vi "执行校准.vi"(3 "校准点位":u16(ring) caption="校准方式：" items=["第一点校准", "第二点校准", "第三点校准"], 5 "校准方式":u16(ring) caption="校准方式：" items=["单点校准", "两点校准", "三点校准"], 6 "校准量程":u16, 7 "校准参数":u16(ring) caption="校准参数：" items=["pH", "DO", "浊度", "电导率", "叶绿素a", "藻密度", "ORP", "COD", "DO2", "氯化物", "氨氮", "水火油"], 8 "error in (no error)":errorcluster caption="错误输入（无错误）", 9 "标液三":cluster{"标准值":dbl, "检测值":dbl, "原始值":dbl} caption="标液三：" {"原始值" format="%#.6f"; "检测值" format="%#.6f"; "标准值" format="%#.6f"}, 10 "标液二":cluster{"标准值":dbl, "检测值":dbl, "原始值":dbl} caption="标液二：" {"原始值" format="%#.6f"; "检测值" format="%#.6f"; "标准值" format="%#.6f"}, 11 "标液一":cluster{"标准值":dbl, "检测值":dbl, "原始值":dbl} caption="标液一：" {"原始值" format="%#.6f"; "检测值" format="%#.6f"; "标准值" format="%#.6f"}) -> (0 "error out":errorcluster)   [LabVIEW 2016, in "斯坦道多参数.lvlib"]
panel:
  in  "选项卡控件":enum32{"选项卡 1"}(tab)
  # "检测值"
  # "原始值"
  # "标准值"
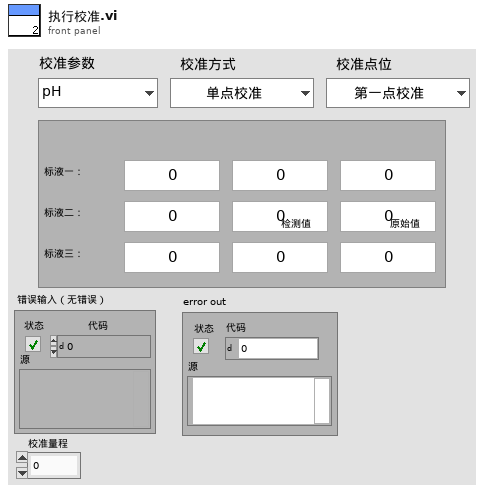
[diagram p1: front panel]
types:
  T1 = typedef "斯坦道多参数.lvlib/探头类型.ctl" = enum16{"禹山", "国弘", "纳清", "STD"}
  T2 = cluster{"pH探头选择":T1, "DO探头选择":T1, "电导率探头选择":T1, "浊度探头选择":T1, "悬浮物探头选择":T1, "叶绿素a探头选择":T1, "蓝绿藻探头选择":T1, "orp探头选择":T1, "COD探头选择":T1, "DO2探头选择":T1, "氨氮探头选择":T1, "水中油探头选择":T1, "余氯探头选择":T1}
  T3 = enum16{"NULL", "pH", "Cond", "DO", "Turb", "ORP", "6", "7", "COD", "9", "氯化物", "11", "12", "13", "14", "15", "16", "水中油"}
  T4 = enum16{"null", "pH", "DO", "浊度", "电导率", "叶绿素a", "藻密度", "氨氮"}
  T5 = enum16{"null", "pH", "DO", "浊度", "电导率", "叶绿素a", "DO2"}
  T6 = enum16{"null", "pH", "DO", "浊度", "电导率", "叶绿素a", "DO2", "藻密度"}
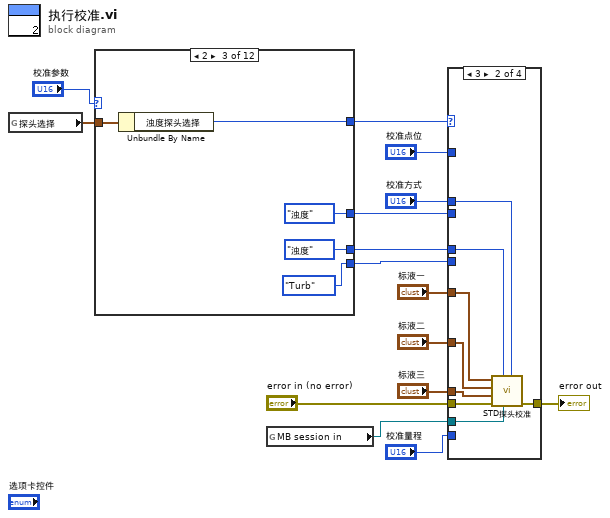
[diagram p0: block diagram]
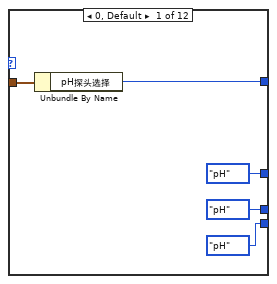
[diagram p2: hidden frame]
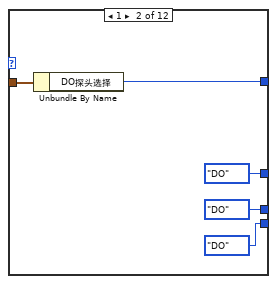
[diagram p3: hidden frame]
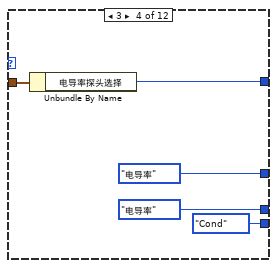
[diagram p4: hidden frame]
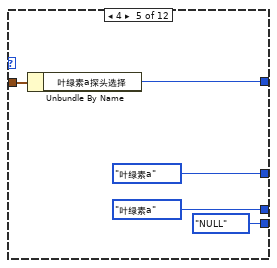
[diagram p5: hidden frame]
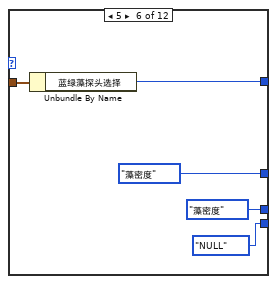
[diagram p6: hidden frame]
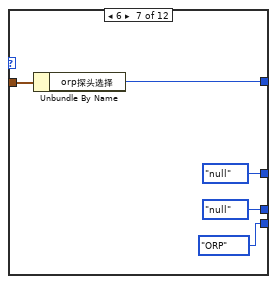
[diagram p7: hidden frame]
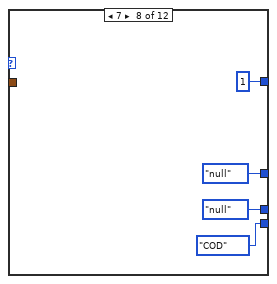
[diagram p8: hidden frame]
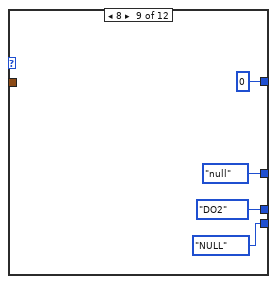
[diagram p9: hidden frame]
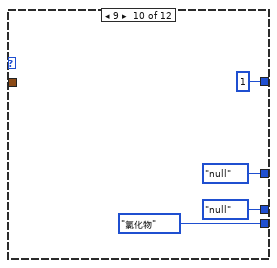
[diagram p10: hidden frame]
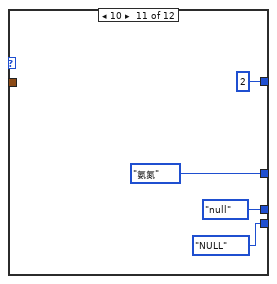
[diagram p11: hidden frame]
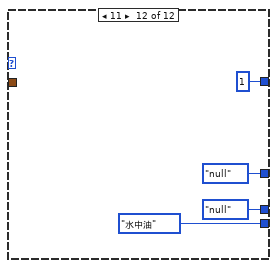
[diagram p12: hidden frame]
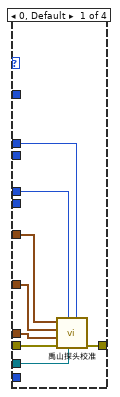
[diagram p13: hidden frame]
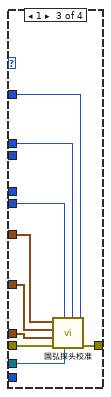
[diagram p14: hidden frame]
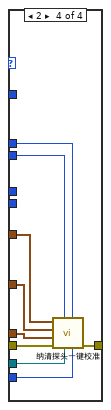
[diagram p15: hidden frame]
diagram:
  n1 = global read "断电保存变量.vi" "探头选择"() -> (w6:T2)
  n2 = case shown="2" "校准参数" {
    tunnel: [T5."pH" ("探头") T5."DO" ("探头") T5."浊度" ("探头") T5."电导率" ("探头") T5."叶绿素a" ("探头") T6."藻密度" ("探头") T5."null" ("探头") T5."null" ("探头") T5."DO2" ("探头") T5."null" ("探头") T5."null" ("探头") T5."null" ("探头")] -> w7
    tunnel: w6 -> [w19 w24 w29 w34 w40 w44 w49 _ _ _ _ _]
    tunnel: [w18 w23 w28 w33 w39 w43 w48 u16 1 ("orp探头选择") u16 0 ("orp探头选择") u16 1 ("orp探头选择") u16 2 ("orp探头选择") u16 1 ("orp探头选择")] -> w5
    tunnel: [T4."pH" ("探头") T4."DO" ("探头") T4."浊度" ("探头") T4."电导率" ("探头") T4."叶绿素a" ("探头") T4."藻密度" ("探头") T4."null" ("探头") T4."null" ("探头") T4."null" ("探头") T4."null" ("探头") T4."氨氮" ("探头") T4."null" ("探头")] -> w4
    tunnel: [T3."pH" ("探头") T3."DO" ("探头") T3."Turb" ("探头") T3."Cond" ("探头") T3."NULL" ("探头") T3."NULL" ("探头") T3."ORP" ("探头") T3."COD" ("探头") T3."NULL" ("探头") T3."氯化物" ("探头") T3."NULL" ("探头") T3."水中油" ("探头")] -> w3
    frame 0, Default {
      n3 = Unbundle By Name(w19) -> ("pH探头选择"=w18:T1)
    }
    frame 1 {
      n4 = Unbundle By Name(w24) -> ("DO探头选择"=w23:T1)
    }
    frame 2 {
      n5 = Unbundle By Name(w29) -> ("浊度探头选择"=w28:T1)
    }
    frame 3 {
      n6 = Unbundle By Name(w34) -> ("电导率探头选择"=w33:T1)
    }
    frame 4 {
      n7 = Unbundle By Name(w40) -> ("叶绿素a探头选择"=w39:T1)
    }
    frame 5 {
      n8 = Unbundle By Name(w44) -> ("蓝绿藻探头选择"=w43:T1)
    }
    frame 6 {
      n9 = Unbundle By Name(w49) -> ("orp探头选择"=w48:T1)
    }
    frame 7 {
    }
    frame 8 {
    }
    frame 9 {
    }
    frame 10 {
    }
    frame 11 {
    }
  }
  n10 = global read "多参数全局变量.vi" "MB session in"() -> (w15:refnum<class "MB_Master.lvclass">)
  n11 = case shown="3" w5 {
    tunnel: w15 -> [w72 w80 w93 w98]
    tunnel: [w78 w86 w94 w104] -> w14
    tunnel: "标液一" -> [w73 w81 w91 w102]
    tunnel: "error in (no error)" -> [w77 w85 w95 w103]
    tunnel: "标液二" -> [w76 w84 w90 w101]
    tunnel: "标液三" -> [w75 w83 w89 w100]
    tunnel: "校准方式" -> [w74 w82 w92 w99]
    tunnel: w7 -> [w71 w79 _ _]
    tunnel: w4 -> [_ _ _ w96]
    tunnel: w3 -> [_ _ w87 _]
    tunnel: "校准点位" -> [_ _ w88 _]
    tunnel: "校准量程" -> [_ _ _ w97]
    frame 0, Default {
      n12 = call "禹山探头校准.vi"("校准方式"=w74, "MB_Master输入"=w72, "探头"=w71, "错误输入（无错误）"=w77, "标液三"=w75, "标液二"=w76, "标液一"=w73) -> ("错误输出"=w78:errorcluster)  [unwired: 4 in]
    }
    frame 3 {
      n13 = call "STD探头校准.vi"("校准方式"=w82, "MB_Master输入"=w80, "探头"=w79, "错误输入（无错误）"=w85, "标液三"=w83, "标液二"=w84, "标液一"=w81) -> ("错误输出"=w86:errorcluster)  [unwired: 4 in]
    }
    frame 1 {
      n14 = call "国弘探头校准.vi"("校准点位"=w88, "校准方式"=w92, "MB_Master输入"=w93, "探头"=w87, "错误输入（无错误）"=w95, "标液三"=w89, "标液二"=w90, "标液一"=w91) -> ("错误输出"=w94:errorcluster)  [unwired: 3 in]
    }
    frame 2 {
      n15 = call "纳清探头一键校准.vi"("校准量程"=w97, "校准方式"=w99, "MB_Master输入"=w98, "探头"=w96, "error in (no error)"=w103, "标液三"=w100, "标液二"=w101, "标液一"=w102) -> ("error out"=w104:errorcluster)  [unwired: 3 in]
    }
  }
  "error out" <- w14
